vi "Start Call (Internal).vi"(4 "Working Directory (default <Not A Path> - System Default)":path=path "" caption="Working Directory", 6 "Event References":T1, 7 "Configuration":refnum<class "configuration.lvclass">, 8 "error in":errorcluster, 9 "Arguments":string[](array[string]), 10 "Exe":string, 11 "Command":string) -> (0 "error out":errorcluster, 3 "New ASE Handle":refnum<class "ase.lvclass">)   [LabVIEW 2024, in "serenial.io-ase.lvlib" / "ase.lvclass"]
doc: "<B>Start an Asynchronous System Executable Call</B>\n\nThe name of an executable should be available in this process's PATH variable. The full path of the executable called will be provided by the \"Did Launch\" User Event.\n\nThe User Events References to generate the \"Did Launch\", \"Standard Output\", \"Standard Error\" and \"Did Exit\" events can be supplied or omitted as required. <B>Ensure that the event registration process for any User Events passed to this VI has already been undertaken</B>.\n\nArguments that are to be passed to the executable are specified in an array. Ensure that each argument specifier or value is in a different array element. E.g. to call the ping executable with the arguments \"-n 10 localhost\" use the element values [ -n, 10, localhost].\n\nThe configuration class allows for override of certain behaviours such as the regular expression used to match the breaks in the Standard Out and Standard Error to be specified.\n\nThis VI generates the following errors:\n-4601: Poorly formatted/incorrect Regular Expression supplied.\n-5691000: Internal Library Error. <Check Error Message for more details>\n-5691301: Unable to launch the executable. <Check Error Message for more details>\n-5691305: Executable name/path parameter cannot be an empty value."
uses:
  ase.lvclass
  Event References.ctl
  Standard Output.ctl
  Standard Error.ctl
  Did Exit.ctl
  configuration/configuration.lvclass
  ase.lvclass/ase.ctl
  Error Internal Library Implementation Error.vi
  <vilib>/Utility/error.llb/Error Cluster From Error Code.vi
  serenial.io-ase.32.dll
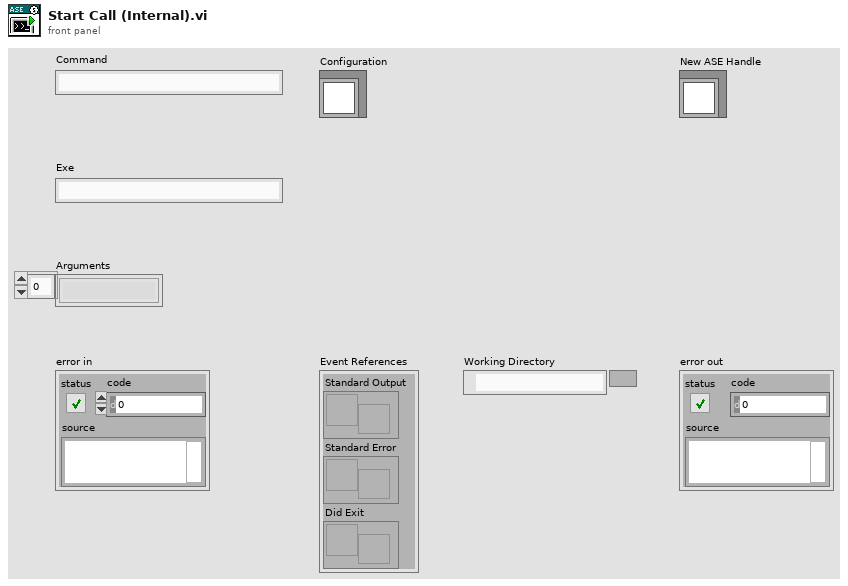
[diagram p1: front panel]
types:
  T1 = typedef "serenial.io-ase.lvlib/ase.lvclass/Event References.ctl" = cluster{"Standard Output":refnum<user-event>, "Standard Error":refnum<user-event>, "Did Exit":refnum<user-event>}
  T2 = cluster{"Stream Split Character Match RegExp Std Out":string, "Stream Split Character Match RegExp Std Err":string}
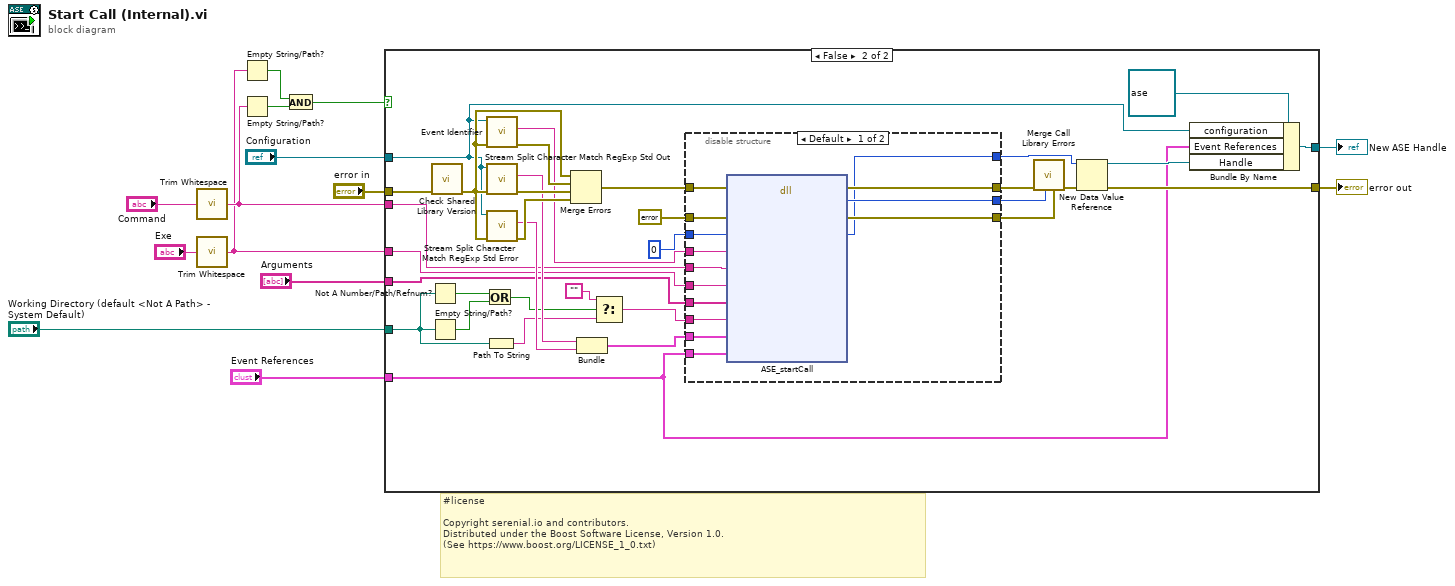
[diagram p0: block diagram]
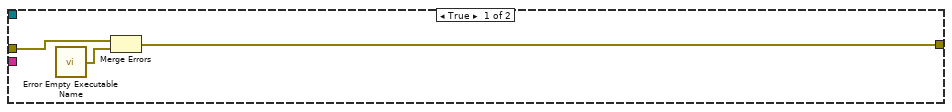
[diagram p2: hidden frame]
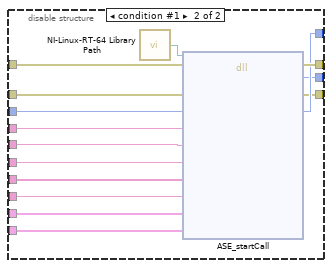
[diagram p3: hidden frame]
diagram:
  # "#license\n\nCopyright serenial.io and contributors.\nDistributed under the Boost Software License, Version 1.0.\n(See https://www.boost.org/LICENSE_1_0.txt)"
  n1 = call "Trim Whitespace.vi"("Input"="Command") -> ("Output"=w3:string)
  n2 = call "Trim Whitespace.vi"("Input"="Exe") -> ("Output"=w2:string)
  n3 = Empty String/Path?(string/path=w2) -> (empty?=w6:bool)
  n4 = Empty String/Path?(string/path=w3) -> (empty?=w5:bool)
  n5 = And(x=w6, y=w5) -> (x .and. y?=w4:bool)
  n6 = case shown="False" w4 {
    tunnel: "error in" -> [w17 w50]
    tunnel: "Working Directory (default <Not A Path> - System Default)" -> [_ w22]
    tunnel: [_ w47] -> w12
    tunnel: "Event References" -> [_ w43]
    tunnel: [w16 w46] -> w10
    tunnel: "Configuration" -> [_ w30]
    tunnel: w3 -> [_ w20]
    tunnel: w2 -> [_ w19]
    tunnel: "Arguments" -> [_ w18]
    frame True {
      n7 = call "Error Empty Executable Name.vi"() -> ("Invalid Executable Name"=w15:errorcluster)
      n8 = Merge Errors(w17, w15) -> (w16:errorcluster)
    }
    frame False {
      n9 = Not A Number/Path/Refnum?(number/path/refnum=w22) -> (NaN/Path/Refnum?=w26:bool)
      n10 = Empty String/Path?(string/path=w22) -> (empty?=w27:bool)
      n11 = call "Check Shared Library Version.vi"("error in"=w50) -> ("error out"=w37:errorcluster)  [unwired: 10 in]
      n12 = Or(x=w26, y=w27) -> (x .or. y?=w25:bool)
      n13 = Path To String(path=w22) -> (string=w23:string)
      n14 = call-dynamic "Event Identifier.vi"("error in (no error)"=w37, "configuration in"=w30) -> ("error out"=w36:errorcluster, "Event Identifier"=w32:string)  [unwired: 8 in]
      n15 = call-dynamic "Stream Split Character Match RegExp Std Out.vi"("error in (no error)"=w37, "configuration in"=w30) -> ("error out"=w35:errorcluster, "Stream Split Character Match RegExp Std Out"=w29:string)  [unwired: 8 in]
      n16 = call-dynamic "Stream Split Character Match RegExp Std Error.vi"("error in (no error)"=w37, "configuration in"=w30) -> ("error out"=w34:errorcluster, "Stream Split Character Match RegExp Std Err"=w28:string)  [unwired: 8 in]
      n17 = Merge Errors(w37, w36, w35, w34) -> (w33:errorcluster)
      n18 = Bundle("Stream Split Character Match RegExp Std Out"=w29, "Stream Split Character Match RegExp Std Err"=w28) -> (w38:T2)  [unwired: 1 in]
      n19 = Select(t="" ("Empty String Constant"), s=w25, f=w23) -> (s? t:f=w21:string)
      n20 = disable-structure "Conditional Disable Structure" shown="Default" {
        disable-tunnel: w33 -> [w64 w79]
        disable-tunnel: errorcluster {"status"=FALSE, "code"=0, "source"=""} ("error in (no error)") -> [w63 w78]
        disable-tunnel: u64 0 ("ASE interface pointer") -> [w62 w77]
        disable-tunnel: w32 -> [w61 w76]
        disable-tunnel: w20 -> [w60 w75]
        disable-tunnel: w38 -> [w59 w73]
        disable-tunnel: w43 -> [w58 w74]
        disable-tunnel: [w57 w72] -> w42
        disable-tunnel: [w56 w70] -> w41
        disable-tunnel: [w55 w69] -> w40
        disable-tunnel: [w54 w71] -> w39
        disable-tunnel: w21 -> [w53 w67]
        disable-tunnel: w19 -> [w52 w66]
        disable-tunnel: w18 -> [w51 w65]
        frame condition #0 (active) {
          n21 = dll-call lib="C:/Users/marc/code/sift-streaming/labview/Sift/Dependencies/asynchronous-system-exec-v2.0.0/serenial.io-ase/ase/serenial.io-ase.*.*" fn="ASE_startCall"(error in=w64, "Error Out"=w63, "ASE interface pointer"=w62, "ID"=w61, "Command"=w60, "Exe"=w52, "Exe-Args"=w51, "Working Directory"=w53, "Stream Split RegEx"=w59, "Even Refs"=w58) -> (error out=w57:errorcluster, "Error Code"=w56:i32, "Error Out"=w55:errorcluster, "ASE interface pointer"=w54:u64)  [unwired: 9 in, 1 out]
        }
        frame condition #1 {
          n22 = call "NI-Linux-RT-64 Library Path.vi"() -> ("Path"=w68:path)
          n23 = dll-call lib="?" fn="ASE_startCall"(path in=w68, error in=w79, "Error Out"=w78, "ASE interface pointer"=w77, "ID"=w76, "cmd"=w75, "exe"=w66, "exe-args"=w65, "Working Directory"=w67, "Stream Split RegEx"=w73, "Even Refs"=w74) -> (error out=w72:errorcluster, "Error Code"=w70:i32, "Error Out"=w69:errorcluster, "ASE interface pointer"=w71:u64)  [unwired: 8 in, 1 out]
        }
      }
      n24 = call "Merge Call Library Errors.vi"("Library Call Returned Error"=w40, "Error Code"=w41, "error in"=w42) -> ("error IO"=w49:errorcluster)  [unwired: 8 in]
      n25 = New Data Value Reference(data value=w39, error in=w49) -> (data value reference=w48:refnum<data-value>, error out=w46:errorcluster)
      n26 = Bundle By Name(cluster=refnum<class "ase.lvclass"> refnum ("serenial.io-ase.lvlib:ase.lvclass"), "configuration"=w30, "Event References"=w43, "Handle"=w48) -> (w47:refnum<class "ase.lvclass">)
    }
  }
  "New ASE Handle" <- w12
  "error out" <- w10
